vi "Test.vi"() -> ()   [LabVIEW 2020, in "allgemeine Sub-VIs.lvlib"]
uses:
  allgemeine Sub-VIs.lvlib
panel:
  out "Y 24":bool
  out "Y 23":bool
  out "Y 22":bool
  out "Y 21":bool
  out "Y 20":bool
  out "Y 19":bool
  out "Y 18":bool
  out "Y 17":bool
  out "Y 16":bool
  out "Y 15":bool
  out "Y 14":bool
  out "Y 13":bool
  in  "Zahl 3":u32
  out "Zahl":u32
  in  "Y 12":bool
  in  "Y 11":bool
  in  "Y 10":bool
  in  "Y 9":bool
  in  "Y 8":bool
  in  "Y 7":bool
  in  "Y 6":bool
  in  "Y 5":bool
  in  "Y 4":bool
  in  "Y 3":bool
  in  "Y 2":bool
  in  "Y 1":bool
  # "Version HP(normal)\nZustand+Anweisungscode               Ventilansteuerungs zahl\nSpülen Filter                                     1 und 3 wechseln\nCalGas                                             4\nMessen 1                                         16      \nCalGasOverflow                                6\nSpülen Leitung 1                               17\nLüften                                               2\nMessen 2                                         32              \nSpülen 2                                           33            \nMessen 3                                         64              \nSpülen 3                                           65           \nMessen 4                                         128             \nSpülen 4                                           129          \nMessen 5                                         256              \nSpülen 5                                           257           \nMessen 6                                         512             \nSpülen 6                                           513"
  # "Version LP\nZustand+Anweisungscode               Ventilansteuerungs zahl\nSpülen Filter                                      1 und 3 wechseln\nCalGas                                             1025\nMessen 1                       VFS2-6        1040      \nCalGasOverflow                                1030 \nSpülen Leitung 1                               17\nLüften                                              2\nMessen 2                                         1056              \nSpülen 2                                           33            \nMessen 3                                         1088              \nSpülen 3                                           65           \nMessen 4                                         1152             \nSpülen 4                                           129          \nMessen 5                                         1280              \nSpülen 5                                           257           \nMessen 6                                         1536             \nSpülen 6                                           513"
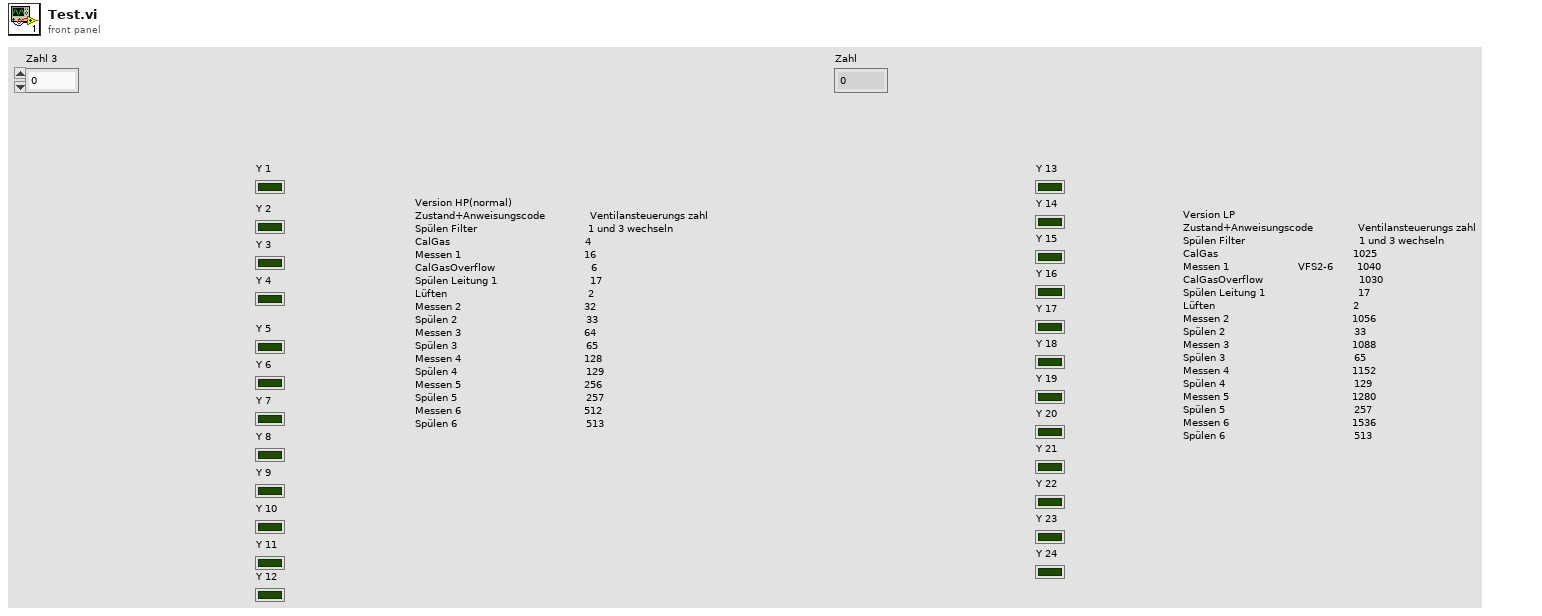
[diagram p1: front panel]
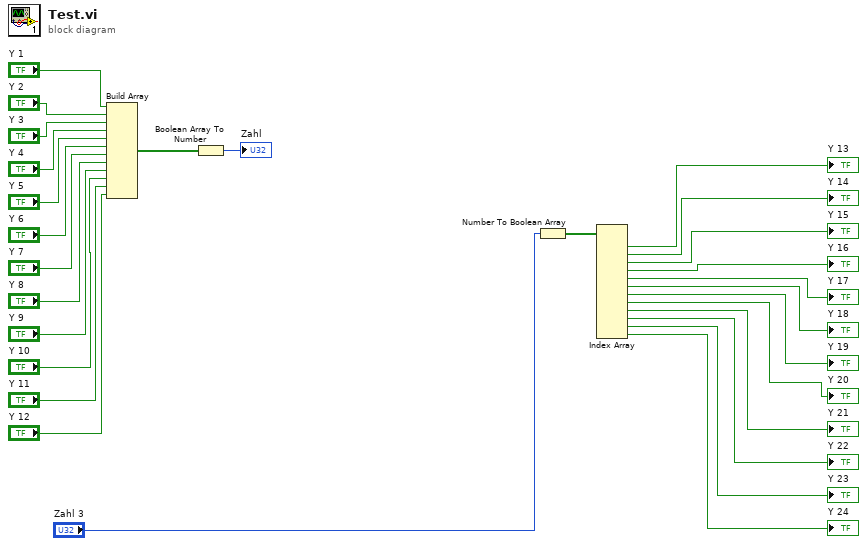
[diagram p0: block diagram]
diagram:
  n1 = Build Array("Y 1", "Y 2", "Y 3", "Y 4", "Y 5", "Y 6", "Y 7", "Y 8", "Y 9", "Y 10", "Y 11", "Y 12") -> (w16:bool[])
  n2 = Boolean Array To Number(Boolean array=w16) -> (number=→"Zahl":u32)
  n3 = Number To Boolean Array(number="Zahl 3") -> (Boolean array=w2:bool[])
  n4 = Index Array(array=w2) -> (element #1=→"Y 13":bool, element #2=→"Y 14":bool, element #3=→"Y 15":bool, element #4=→"Y 16":bool, element #5=→"Y 17":bool, element #6=→"Y 18":bool, element #7=→"Y 19":bool, element #8=→"Y 20":bool, element #9=→"Y 21":bool, element #10=→"Y 22":bool, element #11=→"Y 23":bool, element #12=→"Y 24":bool)  [unwired: 12 in]
